vi "CSM - Read Sessions.vi"(7 "error in (no error)":errorcluster) -> (1 "error out":errorcluster, 2 "Key Found?":bool, 3 "Sections":string[](array[string]))   [LabVIEW 2017, in "INI-Static-Variable-Support.lvlib"]
uses:
  INI-Static-Variable-Support.lvlib
  _fgv-oper.ctl
  <userlib>/_NEVSTOP/Communicable State Machine(CSM)/_Support/ChangeFlag/ChangeFlag-Read.vi
  <userlib>/_NEVSTOP/Communicable State Machine(CSM)/_Support/ChangeFlag/ChangeFlagDB.vi
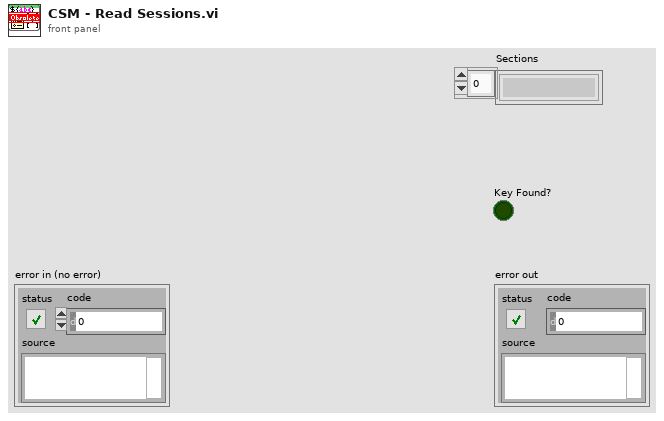
[diagram p1: front panel]
types:
  T1 = typedef "INI-Static-Variable-Support.lvlib/_fgv-oper.ctl" = enum16{"Read", "Write", "Sync", "Sessions", "List Keys", "Load", "List Files", "List Variables", "List Permanent Variables", "Mark Temp Variable as Permenent", "unload", "INIConfig(Memory)", "Reset", "Restore Variable Value"}
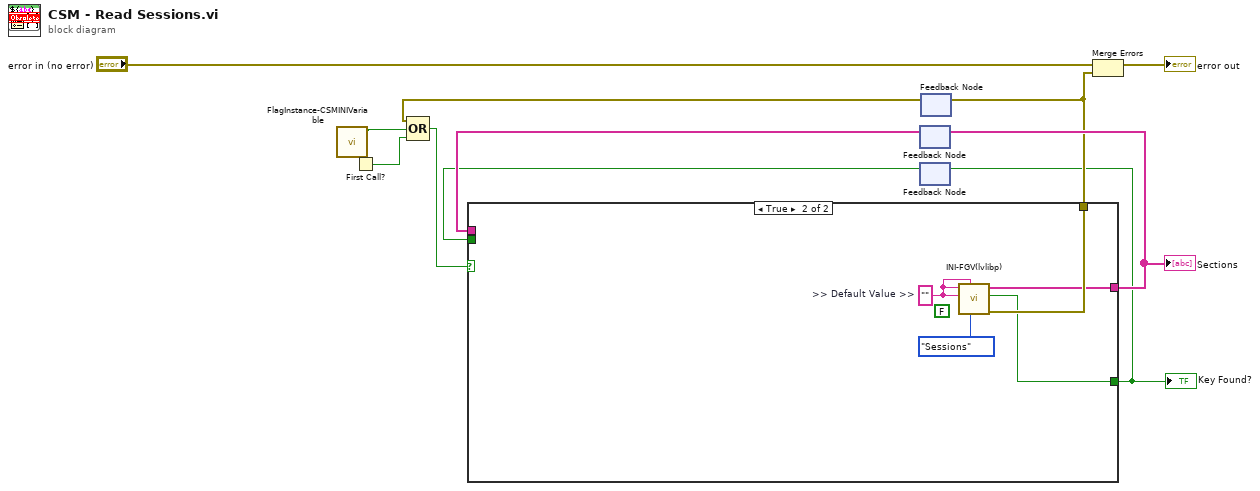
[diagram p0: block diagram]
diagram:
  n1 = call "FlagInstance-CSMINIVariable.vi"() -> ("Changed"=w1:bool)  [unwired: 10 in, 1 out]
  n2 = First Call?() -> (First Call?: T/F=w2:bool)
  n3 = feedback #1() -> (w8:string[])  [unwired: 1 in]
  n4 = feedback #2() -> (w5:bool)  [unwired: 1 in]
  n5 = feedback #3() -> (w4:errorcluster)  [unwired: 1 in]
  n6 = Compound Arithmetic op=OR(w4, w1, w2) -> (w3:bool)
  n7 = case shown="True" w3 {
    tunnel: [_ w17] -> w7
    tunnel: [w13 w16] -> w9
    tunnel: [w12 w15] -> w6
    tunnel: w8 -> [w13 _]
    tunnel: w5 -> [w12 _]
    frame False {
    }
    frame True {
      w14 = ""  # >> Default Value >>
      (unwired) FALSE ("Raw String? (F)")
      n8 = call "INI-FGV(lvlibp).vi"("Enum"=_fgv-oper."Sessions", "Prefered Section"=w14, ">> Default Value >>"=w14, ">> Variable Name >>"=w14) -> ("error out"=w17:errorcluster, "Key?"=w15:bool, "Array"=w16:string[])  [unwired: 4 in, 1 out]
    }
  }
  "Sections" <- w9
  "Key Found?" <- w6
  n9 = feedback-in #1(w9) -> ()
  n10 = feedback-in #2(w6) -> ()
  n11 = feedback-in #3(w7) -> ()
  n12 = Merge Errors("error in (no error)", w7) -> (→"error out":errorcluster)
